vi "LR700 R.vi"(3 "Instrument Address":refnum<visa-resource-name>) -> (0 "Stop":bool, 1 "Measurement":dbl[](array[numeric]) format="%.5e")   [LabVIEW 2020]
doc: "This VI reads the AVS resistance bridge.\nScott Hannahs, NHMFL-FSU, Nov 1993"
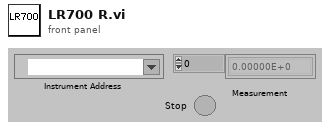
[diagram p1: front panel]
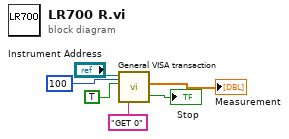
[diagram p0: block diagram]
diagram:
  n1 = call "General VISA transaction.vi"("Wait (mS)"=u32 100 ("wait (mS)"), "Command String"="GET 0", "Eng Units?"=TRUE, "VISA Session"="Instrument Address") -> ("Measurement"=→"Measurement":dbl[], "Stop"=→"Stop":bool)  [unwired: 2 in, 4 out]
